vi "SM_Traffic_Lights_main_IDLE.vi"() -> ()   [LabVIEW 2020]
uses:
  #typedef_Semaphore.ctl
  #typedef_TrafficLights_States.ctl
  #typedef_ProgramData.ctl
  #typedef_Semaphores.ctl
  #typedef_LightTimes.ctl
  #typedef_TimeModes.ctl
  #typedef_TimerAction.ctl
panel:
  in  "Night Mode End":timestamp format="%<%H:%M>T"
  in  "Night Mode Start":timestamp format="%<%H:%M>T"
  in  "stop":bool
  out "West":T1
  out "South":T1
  out "East":T1
  out "North":T1
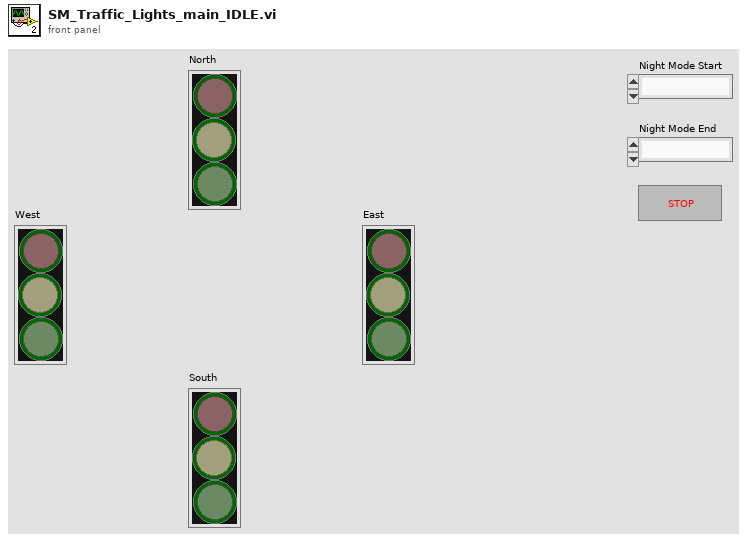
[diagram p1: front panel]
types:
  T1 = typedef "#typedef_Semaphore.ctl" = cluster{"Red":bool, "Yellow":bool, "Green":bool}
  T2 = typedef "#typedef_TrafficLights_States.ctl" = enum16{"Initialize", "Idle", "NS_Green", "NS_Yellow", "NS_Red", "EW_Green", "EW_Yellow", "EW_Red", "NSEW_Yellow_Blink_OFF", "NSEW_Yellow_Blink_ON", "ErrorHandler", "Exit"}
  T3 = typedef "#typedef_TimerAction.ctl" = enum16{"Reset", "TimerElapsed"}
  T4 = typedef "#typedef_ProgramData.ctl" = cluster{"Semaphores":T5, "NextTargetState":T2, "LightTimes":T6, "TimeModes":T7, "CurrentState":T2}
  T5 = typedef "#typedef_Semaphores.ctl" = cluster{"North":T1, "East":T1, "South":T1, "West":T1}
  T6 = typedef "#typedef_LightTimes.ctl" = cluster{"Red (2s)":dbl, "Yellow (2s)":dbl, "Green (5s)":dbl, "Blink ON (2s)":dbl, "Blink OFF (2s)":dbl}
  T7 = typedef "#typedef_TimeModes.ctl" = cluster{"Night Mode Start (23:00)":timestamp, "Night Mode End (06:00)":timestamp}
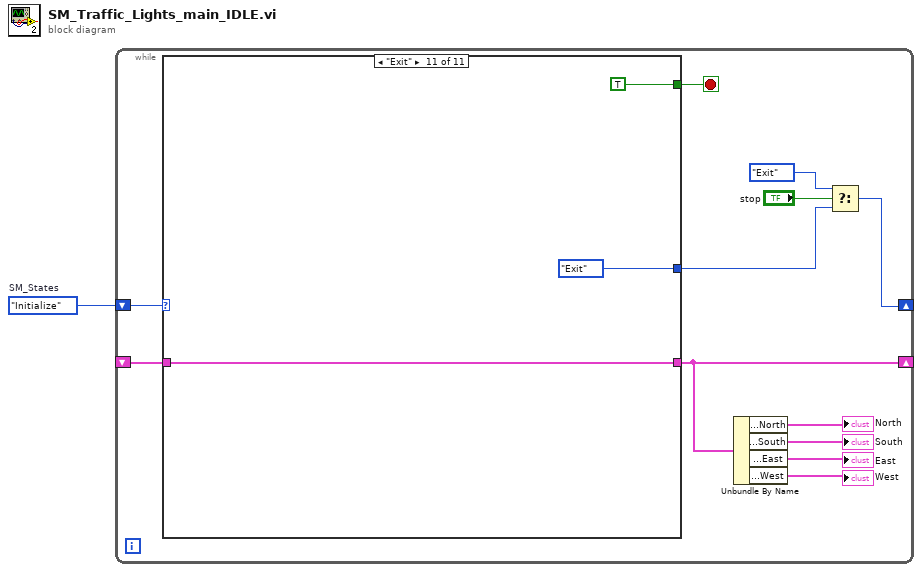
[diagram p0: block diagram]
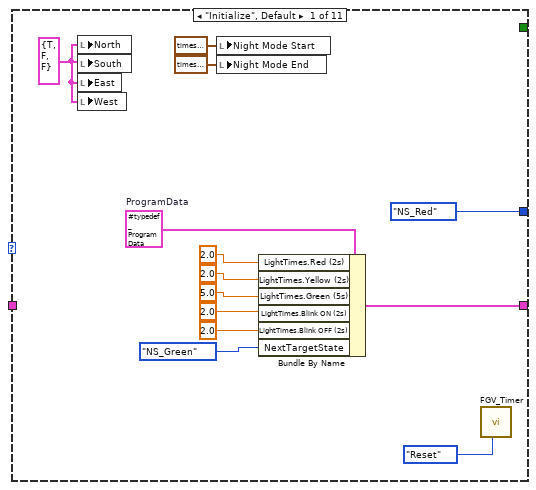
[diagram p2: hidden frame]
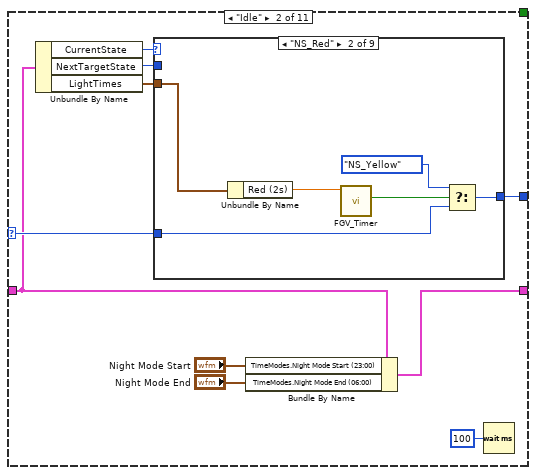
[diagram p3: hidden frame]
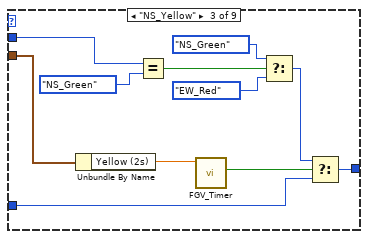
[diagram p5: hidden frame]
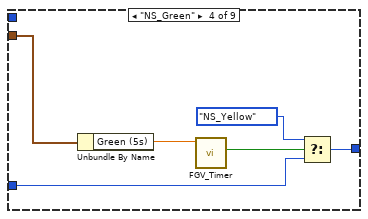
[diagram p6: hidden frame]
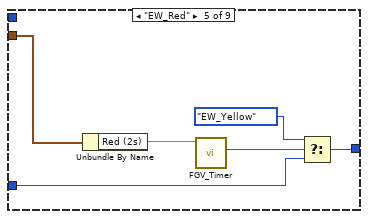
[diagram p7: hidden frame]
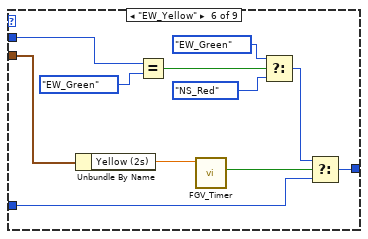
[diagram p8: hidden frame]
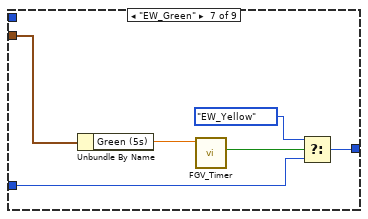
[diagram p9: hidden frame]
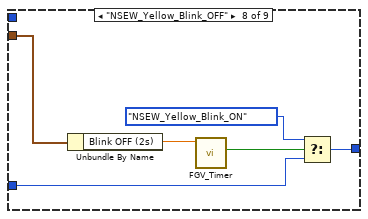
[diagram p10: hidden frame]
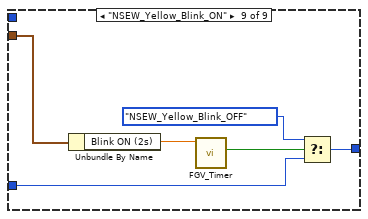
[diagram p11: hidden frame]
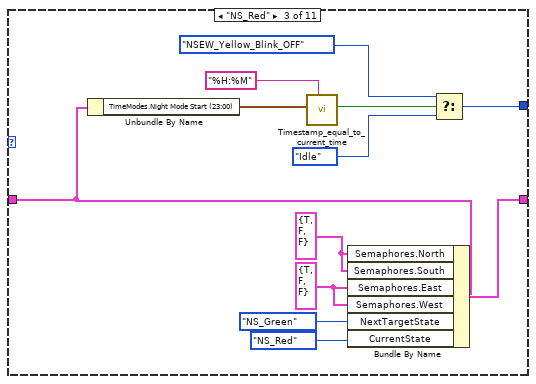
[diagram p12: hidden frame]
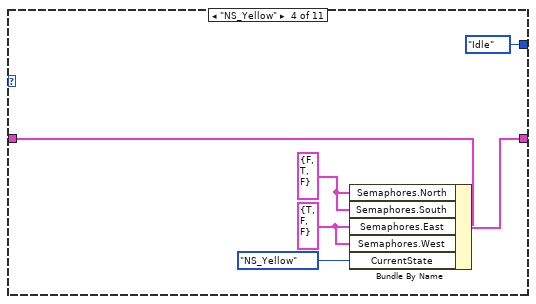
[diagram p13: hidden frame]
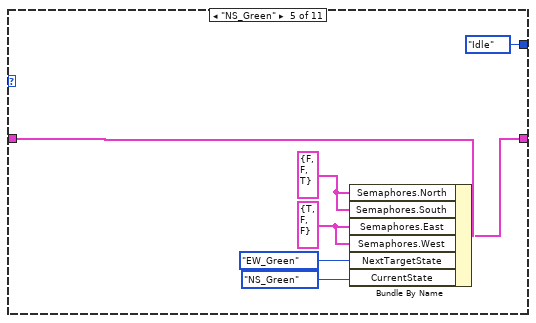
[diagram p14: hidden frame]
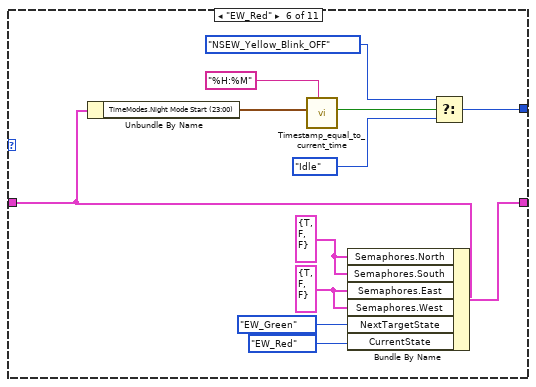
[diagram p15: hidden frame]
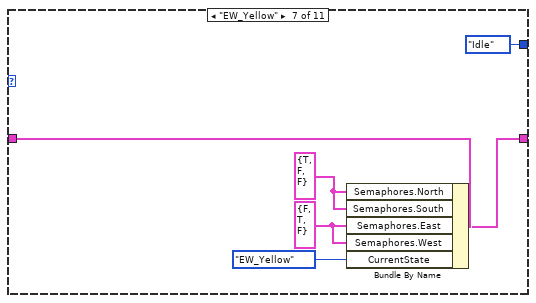
[diagram p16: hidden frame]
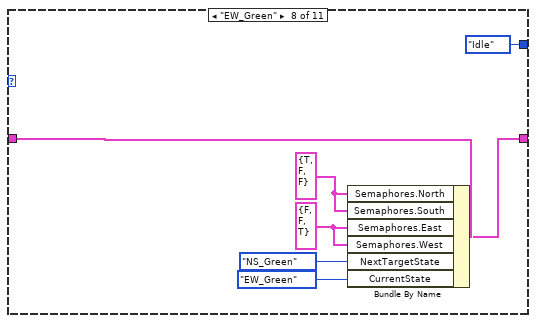
[diagram p17: hidden frame]
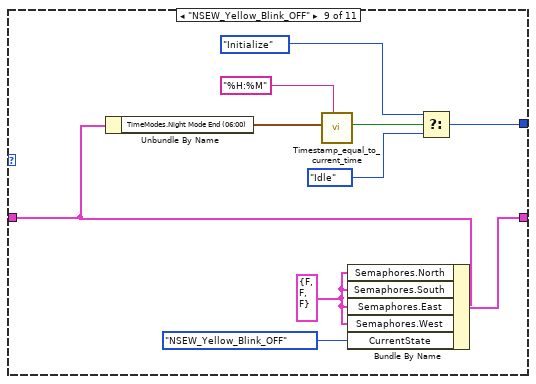
[diagram p18: hidden frame]
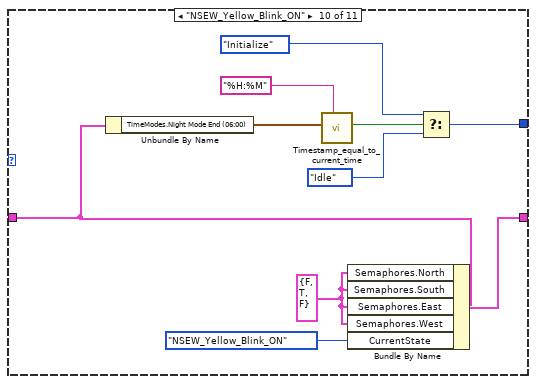
[diagram p19: hidden frame]
diagram:
  w1 = #typedef_TrafficLights_States."Initialize"  # SM_States
  n1 = while {
    shift-right: [w10] -> _
    shift-left: _ -> [w12]
    shift-right: [w2] -> _
    shift-left: w1 -> [w13]
    stop <- w11 stop-if-true
    n2 = case shown="\"Exit\"" w13 {
      selector: w13 -> [_ w33 _ _ _ _ _ _ _ _ _]
      tunnel: [w23 w30 w106 w111 w116 w131 w135 w141 w155 w165 w168] -> w10
      tunnel: w12 -> [_ w31 w103 w110 w117 w128 w136 w142 w149 w159 w168]
      tunnel: [#typedef_TrafficLights_States."NS_Red" ("SM_States") w35 w98 #typedef_TrafficLights_States."Idle" ("SM_States") #typedef_TrafficLights_States."Idle" ("SM_States") w123 #typedef_TrafficLights_States."Idle" ("SM_States") #typedef_TrafficLights_States."Idle" ("SM_States") w148 w158 #typedef_TrafficLights_States."Exit" ("SM_States")] -> w3
      tunnel: [_ _ _ _ _ _ _ _ _ _ TRUE] -> w11
      frame "Initialize", Default {
        w16 = T1 {"Red"=TRUE, "Yellow"=FALSE, "Green"=FALSE} ("North")
        w24 = T4 {"Semaphores"={"North"={"Red"=TRUE, "Yellow"=FALSE, "Green"=FALSE}, "East"={"Red"=TRUE, "Yellow"=FALSE, "Green"=FALSE}, "South"={"Red"=TRUE, "Yellow"=FALSE, "Green"=FALSE}, "West"={"Red"=TRUE, "Yellow"=FALSE, "Green"=FALSE}}, "NextTargetState"=enum."Initialize", "LightTimes"={"Red (2s)"=2.0, "Yellow (2s)"=2.0, "Green (5s)"=5.0, "Blink ON (2s)"=2.0, "Blink OFF (2s)"=2.0}, "TimeModes"={"Night Mode Start (23:00)"=timestamp(0 s since 1904-01-01), "Night Mode End (06:00)"=timestamp(0 s since 1904-01-01)}, "CurrentState"=enum."Initialize"}  # ProgramData
        n3 = local write "North"(w16) -> ()
        n4 = local write "South"(w16) -> ()
        n5 = local write "East"(w16) -> ()
        n6 = local write "West"(w16) -> ()
        n7 = local write "Night Mode Start"(timestamp(79204 s since 1904-01-01) ("Night Mode Start")) -> ()
        n8 = local write "Night Mode End"(timestamp(18000 s since 1904-01-01) ("Night Mode End")) -> ()
        n9 = Bundle By Name(cluster=w24, "LightTimes.Red (2s)"=2.0, "LightTimes.Yellow (2s)"=2.0, "LightTimes.Green (5s)"=5.0, "LightTimes.Blink ON (2s)"=2.0, "LightTimes.Blink OFF (2s)"=2.0, "NextTargetState"=#typedef_TrafficLights_States."NS_Green") -> (w23:T4)
        n10 = call "FGV_Timer.vi"("TimerAction (TimerElapsed)"=#typedef_TimerAction."Reset") -> ()  [unwired: 8 in, 3 out]
      }
      frame "Idle" {
        n11 = Unbundle By Name(w31) -> ("CurrentState"=w36:T2, "NextTargetState"=w34:T2, "LightTimes"=w32:T6)
        n12 = case shown="\"NS_Red\"" w36 {
          tunnel: [w37 w43 w54 w60 w66 w77 w83 w89 w95] -> w35
          tunnel: w34 -> [_ _ w45 _ _ w68 _ _ _]
          tunnel: w33 -> [w37 w40 w52 w57 w63 w75 w80 w86 w92]
          tunnel: w32 -> [_ w38 w50 w55 w61 w73 w78 w84 w90]
          frame "Initialize", Default {
          }
          frame "NS_Red" {
            n13 = Unbundle By Name(w38) -> ("Red (2s)"=w39:dbl)
            n14 = call "FGV_Timer.vi"("TimeToElapse (10) (s)"=w39) -> ("Time Elapsed?"=w41:bool)  [unwired: 8 in, 2 out]
            n15 = Select(t=#typedef_TrafficLights_States."NS_Yellow" ("SM_States"), s=w41, f=w40) -> (s? t:f=w43:T2)
          }
          frame "NS_Yellow" {
            n16 = Unbundle By Name(w50) -> ("Yellow (2s)"=w51:dbl)
            n17 = Equal?(x=w45, y=#typedef_TrafficLights_States."NS_Green" ("SM_States")) -> (x = y?=w48:bool)
            n18 = call "FGV_Timer.vi"("TimeToElapse (10) (s)"=w51) -> ("Time Elapsed?"=w53:bool)  [unwired: 8 in, 2 out]
            n19 = Select(t=#typedef_TrafficLights_States."NS_Green" ("SM_States"), s=w48, f=#typedef_TrafficLights_States."EW_Red" ("SM_States")) -> (s? t:f=w44:T2)
            n20 = Select(t=w44, s=w53, f=w52) -> (s? t:f=w54:T2)
          }
          frame "NS_Green" {
            n21 = Unbundle By Name(w55) -> ("Green (5s)"=w56:dbl)
            n22 = call "FGV_Timer.vi"("TimeToElapse (10) (s)"=w56) -> ("Time Elapsed?"=w58:bool)  [unwired: 8 in, 2 out]
            n23 = Select(t=#typedef_TrafficLights_States."NS_Yellow" ("SM_States"), s=w58, f=w57) -> (s? t:f=w60:T2)
          }
          frame "EW_Red" {
            n24 = Unbundle By Name(w61) -> ("Red (2s)"=w62:dbl)
            n25 = call "FGV_Timer.vi"("TimeToElapse (10) (s)"=w62) -> ("Time Elapsed?"=w64:bool)  [unwired: 8 in, 2 out]
            n26 = Select(t=#typedef_TrafficLights_States."EW_Yellow" ("SM_States"), s=w64, f=w63) -> (s? t:f=w66:T2)
          }
          frame "EW_Yellow" {
            n27 = Unbundle By Name(w73) -> ("Yellow (2s)"=w74:dbl)
            n28 = Equal?(x=w68, y=#typedef_TrafficLights_States."EW_Green" ("SM_States")) -> (x = y?=w71:bool)
            n29 = call "FGV_Timer.vi"("TimeToElapse (10) (s)"=w74) -> ("Time Elapsed?"=w76:bool)  [unwired: 8 in, 2 out]
            n30 = Select(t=#typedef_TrafficLights_States."EW_Green" ("SM_States"), s=w71, f=#typedef_TrafficLights_States."NS_Red" ("SM_States")) -> (s? t:f=w67:T2)
            n31 = Select(t=w67, s=w76, f=w75) -> (s? t:f=w77:T2)
          }
          frame "EW_Green" {
            n32 = Unbundle By Name(w78) -> ("Green (5s)"=w79:dbl)
            n33 = call "FGV_Timer.vi"("TimeToElapse (10) (s)"=w79) -> ("Time Elapsed?"=w81:bool)  [unwired: 8 in, 2 out]
            n34 = Select(t=#typedef_TrafficLights_States."EW_Yellow" ("SM_States"), s=w81, f=w80) -> (s? t:f=w83:T2)
          }
          frame "NSEW_Yellow_Blink_OFF" {
            n35 = Unbundle By Name(w84) -> ("Blink OFF (2s)"=w85:dbl)
            n36 = call "FGV_Timer.vi"("TimeToElapse (10) (s)"=w85) -> ("Time Elapsed?"=w87:bool)  [unwired: 8 in, 2 out]
            n37 = Select(t=#typedef_TrafficLights_States."NSEW_Yellow_Blink_ON" ("SM_States"), s=w87, f=w86) -> (s? t:f=w89:T2)
          }
          frame "NSEW_Yellow_Blink_ON" {
            n38 = Unbundle By Name(w90) -> ("Blink ON (2s)"=w91:dbl)
            n39 = call "FGV_Timer.vi"("TimeToElapse (10) (s)"=w91) -> ("Time Elapsed?"=w93:bool)  [unwired: 8 in, 2 out]
            n40 = Select(t=#typedef_TrafficLights_States."NSEW_Yellow_Blink_OFF" ("SM_States"), s=w93, f=w92) -> (s? t:f=w95:T2)
          }
        }
        n41 = Bundle By Name(cluster=w31, "TimeModes.Night Mode Start (23:00)"="Night Mode Start", "TimeModes.Night Mode End (06:00)"="Night Mode End") -> (w30:T4)
        n42 = Wait (ms)(milliseconds to wait=u32 100) -> ()  [unwired: 1 out]
      }
      frame "NS_Red" {
        w104 = T1 {"Red"=TRUE, "Yellow"=FALSE, "Green"=FALSE} ("Semaphores.North")
        w107 = T1 {"Red"=TRUE, "Yellow"=FALSE, "Green"=FALSE} ("Semaphores.North")
        n43 = Unbundle By Name(w103) -> ("TimeModes.Night Mode Start (23:00)"=w102:timestamp)
        n44 = call "Timestamp_equal_to_current_time.vi"("time format string (%c)"="%H:%M", "time stamp"=w102) -> ("Boolean"=w100:bool)  [unwired: 8 in, 1 out]
        n45 = Bundle By Name(cluster=w103, "Semaphores.North"=w104, "Semaphores.South"=w104, "Semaphores.East"=w107, "Semaphores.West"=w107, "NextTargetState"=#typedef_TrafficLights_States."NS_Green", "CurrentState"=#typedef_TrafficLights_States."NS_Red") -> (w106:T4)
        n46 = Select(t=#typedef_TrafficLights_States."NSEW_Yellow_Blink_OFF" ("SM_States"), s=w100, f=#typedef_TrafficLights_States."Idle" ("SM_States")) -> (s? t:f=w98:T2)
      }
      frame "NS_Yellow" {
        w112 = T1 {"Red"=FALSE, "Yellow"=TRUE, "Green"=FALSE} ("Semaphores.North")
        w113 = T1 {"Red"=TRUE, "Yellow"=FALSE, "Green"=FALSE} ("Semaphores.North")
        n47 = Bundle By Name(cluster=w110, "Semaphores.North"=w112, "Semaphores.South"=w112, "Semaphores.East"=w113, "Semaphores.West"=w113, "CurrentState"=#typedef_TrafficLights_States."NS_Yellow") -> (w111:T4)
      }
      frame "NS_Green" {
        w118 = T1 {"Red"=FALSE, "Yellow"=FALSE, "Green"=TRUE} ("Semaphores.North")
        w120 = T1 {"Red"=TRUE, "Yellow"=FALSE, "Green"=FALSE} ("Semaphores.North")
        n48 = Bundle By Name(cluster=w117, "Semaphores.North"=w118, "Semaphores.South"=w118, "Semaphores.East"=w120, "Semaphores.West"=w120, "NextTargetState"=#typedef_TrafficLights_States."EW_Green", "CurrentState"=#typedef_TrafficLights_States."NS_Green") -> (w116:T4)
      }
      frame "EW_Red" {
        w129 = T1 {"Red"=TRUE, "Yellow"=FALSE, "Green"=FALSE} ("Semaphores.North")
        w132 = T1 {"Red"=TRUE, "Yellow"=FALSE, "Green"=FALSE} ("Semaphores.North")
        n49 = Unbundle By Name(w128) -> ("TimeModes.Night Mode Start (23:00)"=w127:timestamp)
        n50 = call "Timestamp_equal_to_current_time.vi"("time format string (%c)"="%H:%M", "time stamp"=w127) -> ("Boolean"=w125:bool)  [unwired: 8 in, 1 out]
        n51 = Bundle By Name(cluster=w128, "Semaphores.North"=w129, "Semaphores.South"=w129, "Semaphores.East"=w132, "Semaphores.West"=w132, "NextTargetState"=#typedef_TrafficLights_States."EW_Green", "CurrentState"=#typedef_TrafficLights_States."EW_Red") -> (w131:T4)
        n52 = Select(t=#typedef_TrafficLights_States."NSEW_Yellow_Blink_OFF" ("SM_States"), s=w125, f=#typedef_TrafficLights_States."Idle") -> (s? t:f=w123:T2)
      }
      frame "EW_Yellow" {
        w137 = T1 {"Red"=TRUE, "Yellow"=FALSE, "Green"=FALSE} ("Semaphores.North")
        w138 = T1 {"Red"=FALSE, "Yellow"=TRUE, "Green"=FALSE} ("Semaphores.North")
        n53 = Bundle By Name(cluster=w136, "Semaphores.North"=w137, "Semaphores.South"=w137, "Semaphores.East"=w138, "Semaphores.West"=w138, "CurrentState"=#typedef_TrafficLights_States."EW_Yellow") -> (w135:T4)
      }
      frame "EW_Green" {
        w143 = T1 {"Red"=TRUE, "Yellow"=FALSE, "Green"=FALSE} ("Semaphores.North")
        w145 = T1 {"Red"=FALSE, "Yellow"=FALSE, "Green"=TRUE} ("Semaphores.North")
        n54 = Bundle By Name(cluster=w142, "Semaphores.North"=w143, "Semaphores.South"=w143, "Semaphores.East"=w145, "Semaphores.West"=w145, "NextTargetState"=#typedef_TrafficLights_States."NS_Green", "CurrentState"=#typedef_TrafficLights_States."EW_Green") -> (w141:T4)
      }
      frame "NSEW_Yellow_Blink_OFF" {
        w154 = T1 {"Red"=FALSE, "Yellow"=FALSE, "Green"=FALSE} ("Semaphores.North")
        n55 = Unbundle By Name(w149) -> ("TimeModes.Night Mode End (06:00)"=w153:timestamp)
        n56 = call "Timestamp_equal_to_current_time.vi"("time format string (%c)"="%H:%M", "time stamp"=w153) -> ("Boolean"=w151:bool)  [unwired: 8 in, 1 out]
        n57 = Bundle By Name(cluster=w149, "Semaphores.North"=w154, "Semaphores.South"=w154, "Semaphores.East"=w154, "Semaphores.West"=w154, "CurrentState"=#typedef_TrafficLights_States."NSEW_Yellow_Blink_OFF") -> (w155:T4)
        n58 = Select(t=#typedef_TrafficLights_States."Initialize" ("SM_States"), s=w151, f=#typedef_TrafficLights_States."Idle") -> (s? t:f=w148:T2)
      }
      frame "NSEW_Yellow_Blink_ON" {
        w164 = T1 {"Red"=FALSE, "Yellow"=TRUE, "Green"=FALSE} ("Semaphores.North")
        n59 = Unbundle By Name(w159) -> ("TimeModes.Night Mode End (06:00)"=w163:timestamp)
        n60 = call "Timestamp_equal_to_current_time.vi"("time format string (%c)"="%H:%M", "time stamp"=w163) -> ("Boolean"=w161:bool)  [unwired: 8 in, 1 out]
        n61 = Bundle By Name(cluster=w159, "Semaphores.North"=w164, "Semaphores.South"=w164, "Semaphores.East"=w164, "Semaphores.West"=w164, "CurrentState"=#typedef_TrafficLights_States."NSEW_Yellow_Blink_ON") -> (w165:T4)
        n62 = Select(t=#typedef_TrafficLights_States."Initialize" ("SM_States"), s=w161, f=#typedef_TrafficLights_States."Idle") -> (s? t:f=w158:T2)
      }
      frame "Exit" {
      }
    }
    n63 = Unbundle By Name(w10) -> ("Semaphores.North"=→"North":T1, "Semaphores.South"=→"South":T1, "Semaphores.East"=→"East":T1, "Semaphores.West"=→"West":T1)
    n64 = Select(t=#typedef_TrafficLights_States."Exit", s="stop", f=w3) -> (s? t:f=w2:T2)
  }
